vi "measure battery clamp.vi"() -> ()   [LabVIEW 2013]
uses:
  <vilib>/vision/Measure.llb/Edge Options.ctl
  <vilib>/vision/Measure.llb/Edge Polarity.ctl
  <vilib>/vision/NI_Vision_Development_Module.lvlib
panel:
  out "Fitted Circle":T1 {"Average SNR (dB)" format="%.2f"; "Average Strength" format="%.2f"; "Roundness (Real-World)" format="%.2f"; "Radius (Real-World)" format="%.2f"; "Center (Real-World)"."Y" format="%.2f"; "Center (Real-World)"."X" format="%.2f"; "Radius (Pixels)" format="%.2f"; "Center (Pixels)"."Y" format="%.2f"; "Center (Pixels)"."X" format="%.2f"}
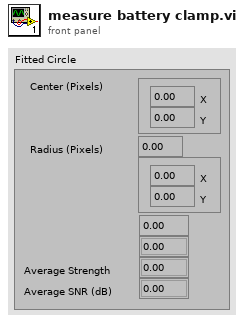
[diagram p1: front panel]
types:
  T1 = cluster{"Center (Pixels)":cluster{"X":sgl, "Y":sgl}, "Radius (Pixels)":dbl, "Center (Real-World)":cluster{"X":sgl, "Y":sgl}, "Radius (Real-World)":dbl, "Roundness (Real-World)":dbl, "Average Strength":dbl, "Average SNR (dB)":dbl}
  T2 = typedef "IMAQ Image.ctl" = refnum<image>
  T3 = cluster{"Algorithm":i32, "Minimum Match Score":sgl, "SubPixel Accuracy":bool, "Rotation Angle Ranges":cluster{"Start":sgl, "End":sgl}[], "Show Search Area":bool, "Show Feature Found":bool, "Show Result":bool}
  T4 = cluster{"Contrast":i32, "Filter width":i32, "Steepness":i32, "Subsampling Ratio":u32, "Show Search Area":bool, "Show Search Lines":bool, "Show Edges Found":bool, "Show Result":bool}
  T5 = typedef "Edge Options.ctl" = cluster{"Edge Polarity":T6, "Kernel Size":u32, "Width":u32, "Minimum Edge Strength":sgl, "Interpolation Type":enum32{"Zero Order", "Bilinear", "Quadratic", "Cubic", "Bilinear Fixed"}, "Data Processing Method":enum32{"Average", "Median"}}
  T6 = typedef "Edge Polarity.ctl" = u32
  T7 = cluster{"Search  Direction":u32, "Edge Options":T5, "Show Search Area":bool, "Show Search Lines":bool, "Show Edges Found":bool, "Show Result":bool, "Search Area Color":u32, "Search Lines Color":u32, "Edge Locations Color":u32, "Result Color":u32, "Overlay Group Name":string}
  T8 = cluster{"Global Rectangle":i32[], "Contours":cluster{"ID":enum32{"External", "Internal"}, "Type":u32, "Coordinates":i32[]}[]}
  T9 = typedef "IMAQ Coordinate System" = cluster{"Reference System":cluster{"Origin":cluster{"X":sgl, "Y":sgl}, "Angle (deg)":sgl, "Axis Reference":u32}, "Measurement System":cluster{"Origin":cluster{"X":sgl, "Y":sgl}, "Angle (deg)":sgl, "Axis Reference":u32}}
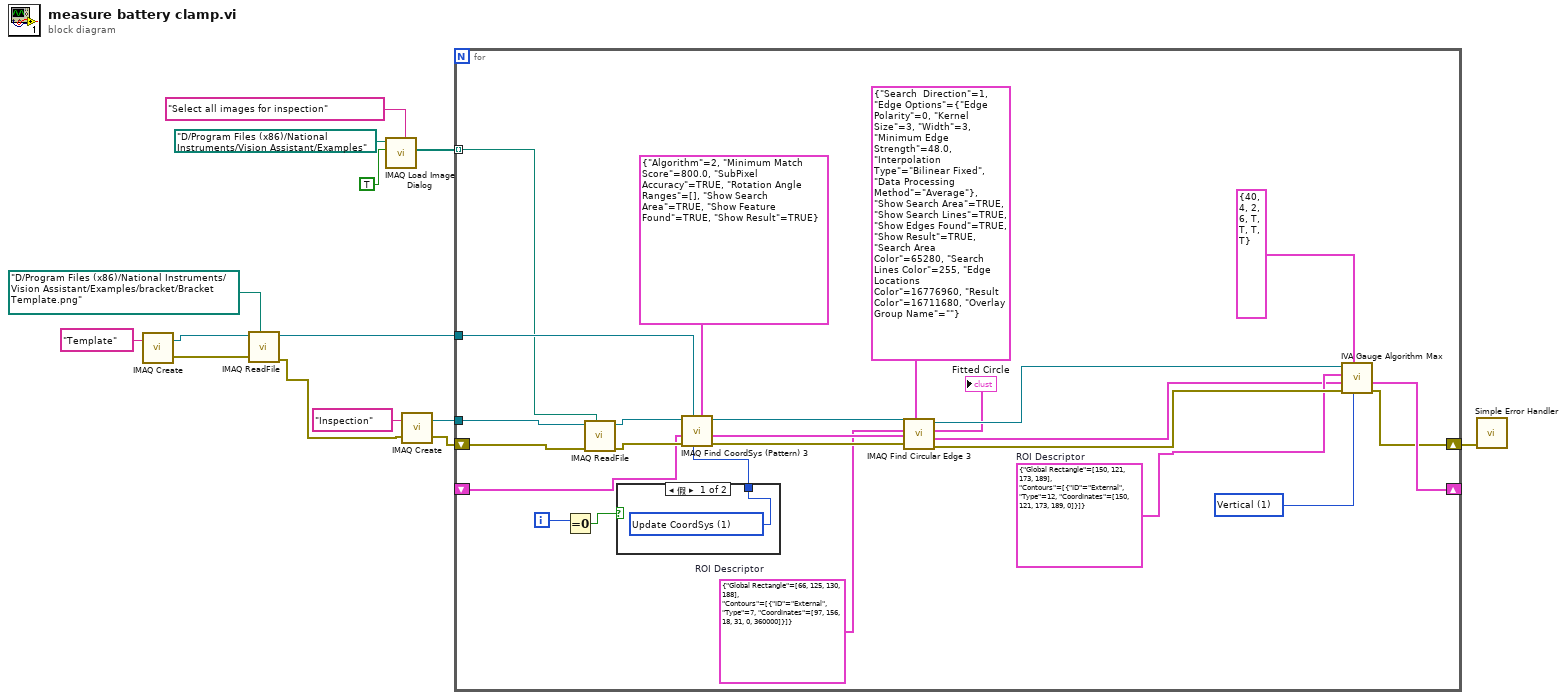
[diagram p0: block diagram]
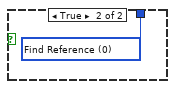
[diagram p2: hidden frame]
diagram:
  n1 = call "IMAQ Create"("Image Name"="Template") -> ("New Image"=w13:T2, "error out"=w12:errorcluster)  [unwired: 4 in]
  n2 = call "IMAQ ReadFile"("File Path"=path "D:/Program Files (x86)/National Instruments/Vision Assistant/Examples/bracket/Bracket Template.png", "error in (no error)"=w12, "Image"=w13) -> ("error out"=w10:errorcluster, "Image Out"=w9:T2)  [unwired: 4 in, 3 out]
  n3 = call "IMAQ Load Image Dialog"("Button Label"="Select all images for inspection", "Multiple Files? (No)"=TRUE, "Start Path"=path "D:/Program Files (x86)/National Instruments/Vision Assistant/Examples") -> ("Paths"=w5:path[])  [unwired: 6 in, 2 out]
  n4 = call "IMAQ Create"("Image Name"="Inspection", "error in (no error)"=w10) -> ("New Image"=w8:T2, "error out"=w7:errorcluster)  [unwired: 3 in]
  n5 = for {
    shift-right: [w19] -> w2
    shift-left: w7 -> [w31]
    shift-right: [w20] -> _
    shift-left: _ -> [w18]
    tunnel: w9 -> [w29]
    tunnel: w8 -> [w30]
    tunnel: w5 -> [w23] mode=indexing
    i -> [w27]
    w17 = T8 {"Global Rectangle"=[66, 125, 130, 188], "Contours"=[{"ID"=enum."External", "Type"=7, "Coordinates"=[97, 156, 18, 31, 0, 360000]}]}  # ROI Descriptor
    w35 = u32 1 items=["Horizontal", "Vertical"] ("Scanning axis")
    w34 = T8 {"Global Rectangle"=[150, 121, 173, 189], "Contours"=[{"ID"=enum."External", "Type"=12, "Coordinates"=[150, 121, 173, 189, 0]}]}  # ROI Descriptor
    n6 = Equal To 0?(x=w27) -> (x = 0?=w26:bool)
    n7 = call "IMAQ ReadFile"("File Path"=w23, "error in (no error)"=w31, "Image"=w30) -> ("error out"=w25:errorcluster, "Image Out"=w22:T2)  [unwired: 4 in, 3 out]
    n8 = case shown="假" w26 {
      tunnel: [w40 w41] -> w28
      frame False {
        w40 = u16 1 items=["Find Reference", "Update CoordSys"] ("Mode")
      }
      frame True {
        w41 = u16 0 items=["Find Reference", "Update CoordSys"] ("Mode")
      }
    }
    n9 = call "IMAQ Find CoordSys (Pattern) 3"("Settings"=T3 {"Algorithm"=2, "Minimum Match Score"=800.0, "SubPixel Accuracy"=TRUE, "Rotation Angle Ranges"=[], "Show Search Area"=TRUE, "Show Feature Found"=TRUE, "Show Result"=TRUE}, "Mode"=w28, "Template"=w29, "error in"=w25, "Coordinate System In"=w18, "Image"=w22) -> ("error out"=w33:errorcluster, "Coordinate System Out"=w21:T9, "Image Out"=w32:T2)  [unwired: 1 in, 2 out]
    n10 = call "IMAQ Find Circular Edge 3"("Options"=T7 {"Search  Direction"=1, "Edge Options"={"Edge Polarity"=0, "Kernel Size"=3, "Width"=3, "Minimum Edge Strength"=48.0, "Interpolation Type"=enum."Bilinear Fixed", "Data Processing Method"=enum."Average"}, "Show Search Area"=TRUE, "Show Search Lines"=TRUE, "Show Edges Found"=TRUE, "Show Result"=TRUE, "Search Area Color"=65280, "Search Lines Color"=255, "Edge Locations Color"=16776960, "Result Color"=16711680, "Overlay Group Name"=""}, "error in (no error)"=w33, "Coordinate System"=w21, "ROI Descriptor"=w17, "Image"=w32) -> ("error out"=w39:errorcluster, "Coordinate System (duplicate)"=w15:T9, "Fitted Circle"=→"Fitted Circle":T1, "Image Out"=w37:T2)  [unwired: 2 in, 1 out]
    n11 = call <vilib>:"IVA Gauge Algorithm Max.vi"("Scanning axis"=w35, "Settings"=T4 {"Contrast"=40, "Filter width"=4, "Steepness"=2, "Subsampling Ratio"=6, "Show Search Area"=TRUE, "Show Search Lines"=TRUE, "Show Edges Found"=TRUE, "Show Result"=TRUE}, "error in (no error)"=w39, "Coordinate System"=w15, "ROI Descriptor"=w34, "Image"=w37) -> ("error out"=w19:errorcluster, "Coordinate System (duplicate)"=w20:T9)  [unwired: 4 out]
  }
  n12 = call <vilib>:"Simple Error Handler.vi"("error in (no error)"=w2) -> ()  [unwired: 4 in, 5 out]
